vi "rotate V1.2.vi"(8 "error in (no error)":errorcluster, 10 "speed":dbl=100.0 format="%#_13g", 11 "degree":dbl) -> (0 "error out":errorcluster)   [LabVIEW 2019]
uses:
  <vilib>/Platform/TimedLoop/XDataNode/timing_clust.ctl
  <vilib>/Platform/TimedLoop/XDataNode/nitl_modes.ctl
  <vilib>/Platform/TimedLoop/XDataNode/wakeup.ctl
  <vilib>/platform/TimedLoop/XDataNode/XDataNode.xnode
  <vilib>/Platform/TimedLoop/XDataNode/XDNodeRunTimeDep.lvlib
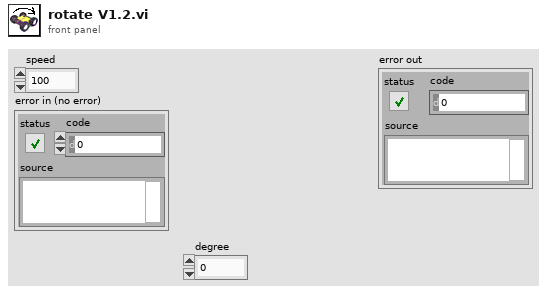
[diagram p1: front panel]
types:
  T1 = typedef "XDNodeRunTimeDep.lvlib/timing_clust.ctl" = cluster{"Expected End [f-1]":u64, "Actual End [f-1]":u64, "Finished Late? [f-1]":bool, "Expected End [i-1]":u64, "Actual End [i-1]":u64, "Finished Late? [i-1]":bool, "Expected Start [i]":u64, "Actual Start [i]":u64, "Expected Start [f]":u64, "Actual Start [f]":u64, "Source Name":string, "Structure Name":string, "Period":i64, "Deadline":i64, "Offset":i64, "Start":i64, "Priority":i32, "Timeout":i32, "Mode":T2, "Wakeup Reason":T3, "Error":errorcluster, "Source Type":string, "Secondary Source Type":string, "Global End Time":u64, "Global Start Time":u64, "Frame Duration":u64, "Iteration Duration":u64, "Assigned CPU":i32, "I/O Scan Engine Mode":u32}
  T2 = typedef "XDNodeRunTimeDep.lvlib/nitl_modes.ctl" = enum32{"No Change", "Process missed periods, maintain original phase", "Discard missed periods, maintain original phase", "Process missed periods, ignore original phase", "Discard missed periods, ignore original phase"}
  T3 = typedef "XDNodeRunTimeDep.lvlib/wakeup.ctl" = enum32{"Normal", "Aborted", "Asynchronous wakeup", "Timing source error", "Timed loop error", "Timeout"}
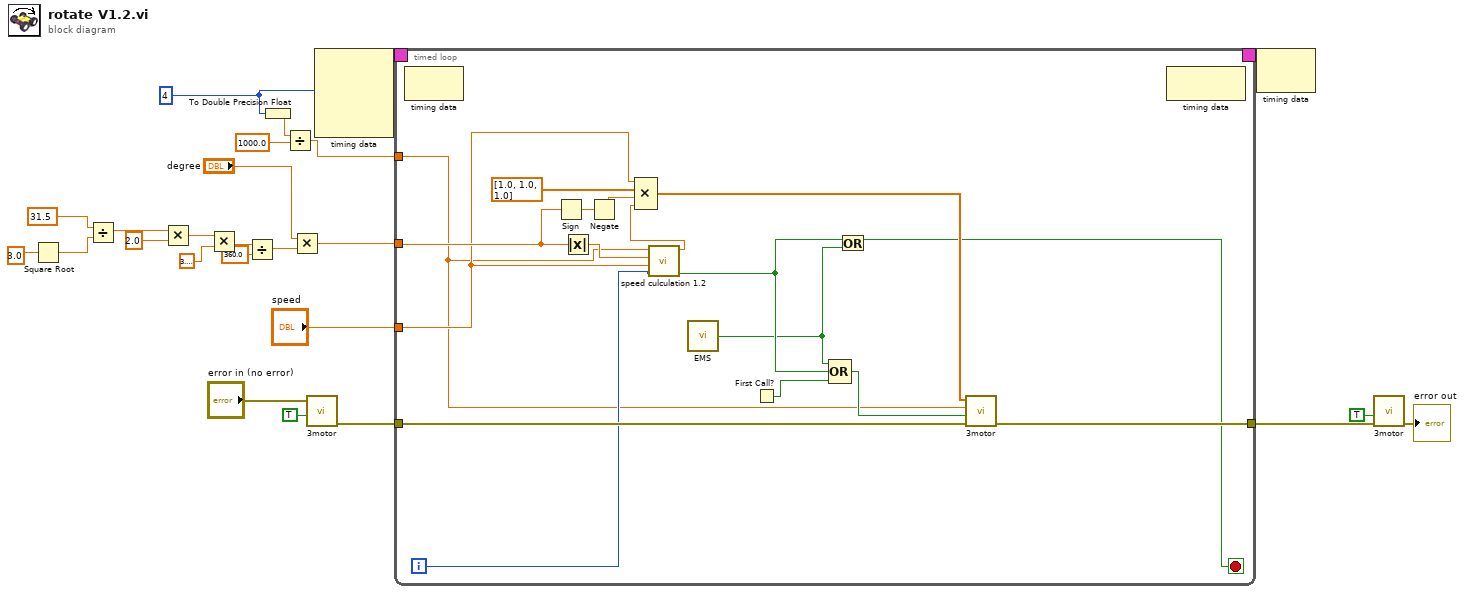
[diagram p0: block diagram]
diagram:
  w11 = i64 4 ("Period")
  n1 = Square Root(x=3.0) -> (sqrt(x)=w24:dbl)
  n2 = Divide(x=31.5, y=w24) -> (x/y=w22:dbl)
  n3 = Multiply(x=w22, y=2.0) -> (x*y=w19:dbl)
  n4 = Multiply(x=w19, y=3.141592653589793) -> (x*y=w18:dbl)
  n5 = Divide(x=w18, y=360.0) -> (x/y=w16:dbl)
  n6 = To Double Precision Float(number=w11) -> (double precision float=w10:dbl)
  n7 = Divide(x=w10, y=1000.0) -> (x/y=w8:dbl)
  n8 = Multiply(x="degree", y=w16) -> (x*y=w12:dbl)
  n9 = call "3motor.vi"("error in (no error)"="error in (no error)", "Reset"=TRUE) -> ("error out"=w6:errorcluster)  [unwired: 8 in, 1 out]
  n10 = node-c288(w11) -> (w14:T1)  [unwired: 3 in]
  n11 = timed-loop {
    timing: w14 -> [_]
    timing-out: [_] -> w13
    tunnel: w12 -> [w40]
    tunnel: w8 -> [w31]
    tunnel: "speed" -> [w33]
    tunnel: w6 -> [w42]
    tunnel: [w41] -> w5
    i -> [w34]
    stop <- w27 stop-if-true
    n12 = node-c288() -> ()  [unwired: 1 in, 1 out]
    n13 = Sign(1:w40) -> (0:w39:dbl)
    n14 = Absolute Value(x=w40) -> (abs(x)=w32:dbl)
    n15 = Negate(x=w39) -> (-x=w28:dbl)
    n16 = call "speed culculation 1.2.vi"("i"=w34, "Speed(RPM)"=w33, "distance"=w32, "dt(s)"=w31) -> ("complet?"=w30:bool, "Speed"=w29:dbl)  [unwired: 4 in, 2 out]
    n17 = Compound Arithmetic op=MULTIPLY(w33, dbl[] [1.0, 1.0, 1.0], w28, w29) -> (w37:dbl[])
    n18 = call "EMS.vi"() -> ("A/DIO4 (Pin 19)"=w26:bool)
    n19 = First Call?() -> (First Call?: T/F=w36:bool)
    n20 = Compound Arithmetic op=OR(w26, w30, w36) -> (w35:bool)
    n21 = Or(x=w30, y=w26) -> (x .or. y?=w27:bool)
    n22 = call "3motor.vi"("error in (no error)"=w42, "Reset"=w35, "dt(s)"=w31, "Motor speed"=w37) -> ("error out"=w41:errorcluster)  [unwired: 6 in, 1 out]
    n23 = node-c288() -> ()  [unwired: 1 in, 1 out]
  }
  n24 = node-c288(w13) -> ()  [unwired: 1 out]
  n25 = call "3motor.vi"("error in (no error)"=w5, "Reset"=TRUE) -> ("error out"=→"error out":errorcluster)  [unwired: 8 in, 1 out]
